vi "Agilent U2000 Series Acquire Measurement.vi"() -> ()   [LabVIEW 2018]
doc: "This example shows how to acquire a power measurement using the VIs of the driver.\n\nNote:\nThis example is not applicable for U2021/2XA."
uses:
  Agilent U2000 Series.lvlib
panel:
  in  "Timeout (10000 ms)":u32=10000
  out "Measurement":dbl
  in  "VISA resource name":refnum<visa-resource-name>
  # "(c) 2011-2015 National Instruments.  ALL RIGHTS RESERVED."
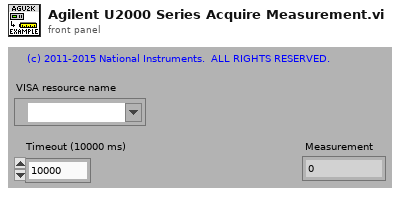
[diagram p1: front panel]
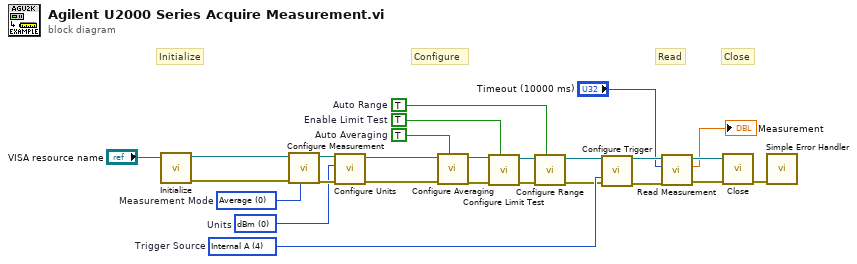
[diagram p0: block diagram]
diagram:
  w16 = 4 items=["Bus", "External", "Hold", "Immediate", "Internal A"]  # Trigger Source
  w17 = 0 items=["Average", "Normal"]  # Measurement Mode
  w9 = TRUE  # Enable Limit Test
  w18 = u16 0 items=["dBm", "W"]  # Units
  w10 = TRUE  # Auto Averaging
  w8 = TRUE  # Auto Range
  # "Close"
  # "Read"
  # "Configure"
  # "Initialize"
  n1 = call "Initialize.vi"("VISA resource name"="VISA resource name") -> ("error out"=w21:errorcluster, "VISA resource name out"=w22:refnum<visa-resource-name>)  [unwired: 3 in, 6 out]
  n2 = call "Configure Measurement.vi"("Measurement Function (0: Average)"=w17, "error in (no error)"=w21, "VISA resource name"=w22) -> ("error out"=w19:errorcluster, "VISA resource name out"=w20:refnum<visa-resource-name>)  [unwired: 7 in]
  n3 = call "Configure Units.vi"("error in (no error)"=w19, "Units (0: dBm)"=w18, "VISA resource name"=w20) -> ("error out"=w13:errorcluster, "VISA resource name out"=w14:refnum<visa-resource-name>)  [unwired: 1 in, 6 out]
  n4 = call "Configure Averaging.vi"("Enable Averaging (T: Enable)"=w10, "error in (no error)"=w13, "VISA resource name"=w14) -> ("error out"=w11:errorcluster, "VISA resource name out"=w12:refnum<visa-resource-name>)  [unwired: 7 in]
  n5 = call "Configure Limit Test.vi"("Limit Test (T: Enable)"=w9, "error in (no error)"=w11, "VISA resource name"=w12) -> ("error out"=w6:errorcluster, "VISA resource name out"=w7:refnum<visa-resource-name>)  [unwired: 2 in, 5 out]
  n6 = call "Configure Range.vi"("Auto Range (T: Enable)"=w8, "error in (no error)"=w6, "VISA resource name"=w7) -> ("error out"=w5:errorcluster, "VISA resource name out"=w15:refnum<visa-resource-name>)  [unwired: 7 in]
  n7 = call "Configure Trigger.vi"("VISA resource name"=w15, "Trigger Source (3: Immediate)"=w16, "error in (no error)"=w5) -> ("VISA resource name out"=w24:refnum<visa-resource-name>, "error out"=w25:errorcluster)  [unwired: 5 in, 6 out]
  n8 = call "Read Measurement.vi"("error in (no error)"=w25, "Timeout (10000 ms)"="Timeout (10000 ms)", "VISA resource name"=w24) -> ("error out"=w3:errorcluster, "Measurement"=→"Measurement":dbl, "VISA resource name out"=w4:refnum<visa-resource-name>)  [unwired: 6 out]
  n9 = call "Close.vi"("error in (no error)"=w3, "VISA resource name"=w4) -> ("error out"=w23:errorcluster)  [unwired: 9 out]
  n10 = call <vilib>:"Simple Error Handler.vi"("error in (no error)"=w23) -> ()  [unwired: 1 in, 8 out]
